vi "Save Section Datas.vi"(8 "error in (no error)":errorcluster, 11 "Section in":refnum<data-value>) -> (0 "error out":errorcluster, 2 "Data":string, 3 "Section out":refnum<data-value>)   [LabVIEW 2013, in "Hierarchy Framework.lvlib" / "Section.lvclass"]
uses:
  Section.lvclass
  Item/Item.lvclass
  Channel/Channel.lvclass
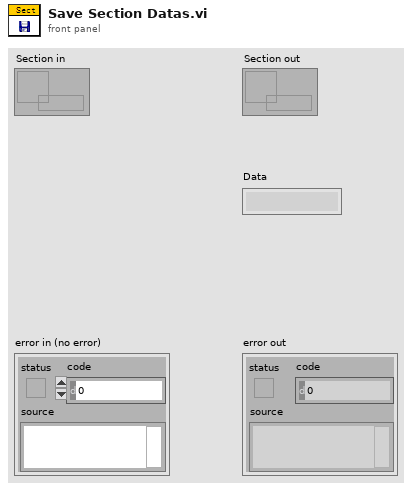
[diagram p1: front panel]
types:
  T1 = typedef "Hierarchy Framework.lvlib/Channel.lvclass/Dimensions.ctl" = cluster{"Row":i32, "Column":i32}
  T2 = typedef "Hierarchy Framework.lvlib/Channel.lvclass/IOType.ctl" = enum16{"Input", "Output"}
  T3 = typedef "Hierarchy Framework.lvlib/Channel.lvclass/Type.ctl" = enum16{"S_Channel", "S_M_Parameter", "S_M_Signal"}
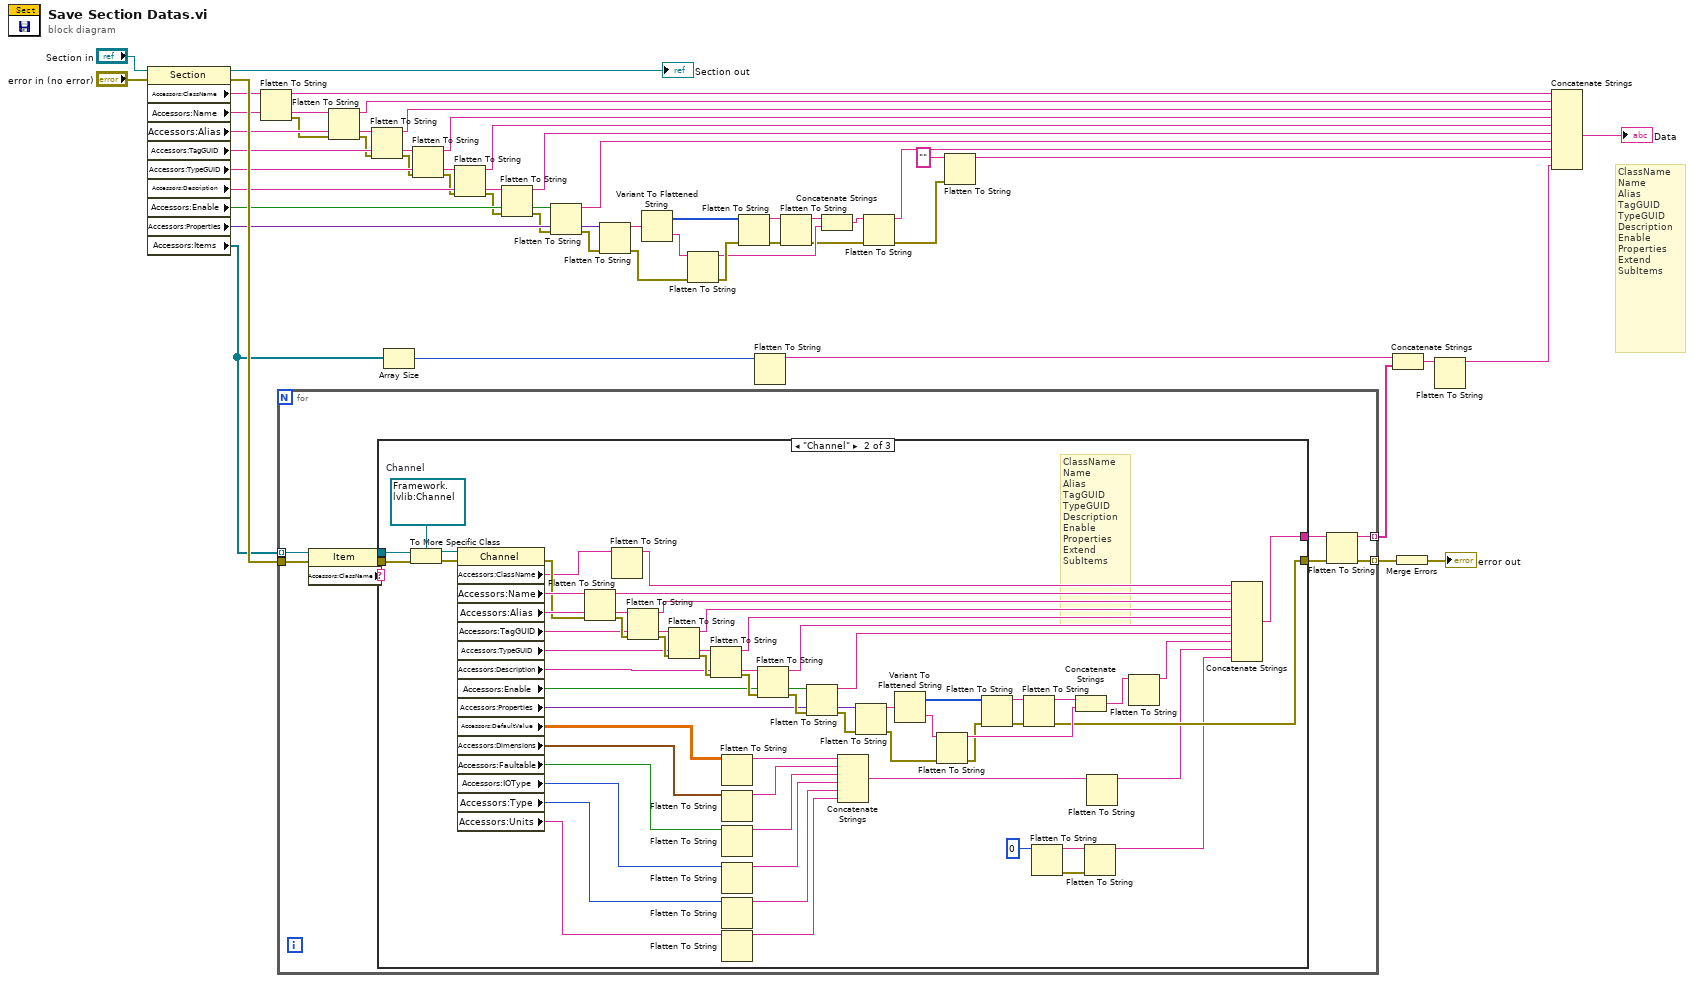
[diagram p0: block diagram]
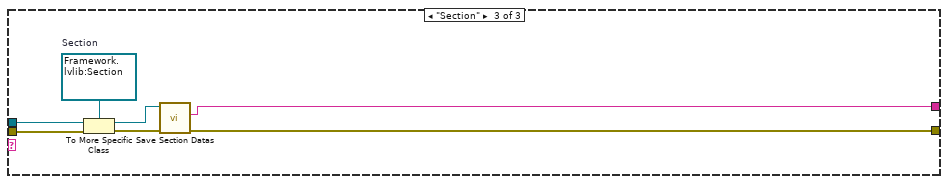
[diagram p3: hidden frame]
diagram:
  # "ClassName\nName\nAlias\nTagGUID\nTypeGUID\nDescription\nEnable\nProperties\nExtend\nSubItems"
  n1 = property class="Section"(reference="Section in", error in="error in (no error)") -> (reference out=→"Section out":refnum<data-value>, error out=w45:errorcluster, "Accessors:ClassName"=w11:string, "Accessors:Name"=w44:string, "Accessors:Alias"=w43:string, "Accessors:TagGUID"=w42:string, "Accessors:TypeGUID"=w41:string, "Accessors:Description"=w40:string, "Accessors:Enable"=w34:bool, "Accessors:Properties"=w30:variant, "Accessors:Items"=w16:refnum<data-value>[])
  n2 = Flatten To String(anything=w11) -> (data string=w9:string, error out=w10:errorcluster)  [unwired: 3 in, 1 out]
  n3 = for {
    tunnel: w16 -> [w59] mode=indexing
    tunnel: [w51] -> w49 mode=indexing
    tunnel: w45 -> [w56]
    tunnel: [w54] -> w12 mode=indexing
    n4 = property class="Item"(reference=w59, error in=w56) -> (reference out=w58:refnum<data-value>, error out=w57:errorcluster, "Accessors:ClassName"=w55:string)
    n5 = case shown="\"Channel\"" w55 {
      tunnel: w58 -> [_ w118 w125]
      tunnel: w57 -> [w60 w117 w124]
      tunnel: [_ w72 w120] -> w53
      tunnel: [w60 w71 w119] -> w52
      frame Default {
      }
      frame "Channel" {
        w116 = refnum<data-value> refnum  # Channel
        # "ClassName\nName\nAlias\nTagGUID\nTypeGUID\nDescription\nEnable\nProperties\nExtend\nSubItems"
        n6 = To More Specific Class(target class=w116, reference=w118, error in=w117) -> (specific class reference=w87:refnum<data-value>, error out=w88:errorcluster)
        n7 = property class="Channel"(reference=w87, error in=w88) -> (error out=w83:errorcluster, "Accessors:ClassName"=w62:string, "Accessors:Name"=w89:string, "Accessors:Alias"=w90:string, "Accessors:TagGUID"=w91:string, "Accessors:TypeGUID"=w92:string, "Accessors:Description"=w93:string, "Accessors:Enable"=w98:bool, "Accessors:Properties"=w102:variant, "Accessors:DefaultValue"=w86:dbl[][], "Accessors:Dimensions"=w84:T1, "Accessors:Faultable"=w85:bool, "Accessors:IOType"=w81:T2, "Accessors:Type"=w80:T3, "Accessors:Units"=w82:string)  [unwired: 1 out]
        n8 = Flatten To String(anything=w89, error in (no error)=w83) -> (data string=w79:string, error out=w110:errorcluster)  [unwired: 2 in, 1 out]
        n9 = Flatten To String(anything=w62) -> (data string=w70:string)  [unwired: 3 in, 2 out]
        n10 = Flatten To String(anything=w90, error in (no error)=w110) -> (data string=w94:string, error out=w111:errorcluster)  [unwired: 2 in, 1 out]
        n11 = Flatten To String(anything=w91, error in (no error)=w111) -> (data string=w95:string, error out=w112:errorcluster)  [unwired: 2 in, 1 out]
        n12 = Flatten To String(anything=w92, error in (no error)=w112) -> (data string=w96:string, error out=w113:errorcluster)  [unwired: 2 in, 1 out]
        n13 = Flatten To String(anything=w86) -> (data string=w78:string)  [unwired: 3 in, 2 out]
        n14 = Flatten To String(anything=w84) -> (data string=w77:string)  [unwired: 3 in, 2 out]
        n15 = Flatten To String(anything=w85) -> (data string=w76:string)  [unwired: 3 in, 2 out]
        n16 = Flatten To String(anything=w81) -> (data string=w75:string)  [unwired: 3 in, 2 out]
        n17 = Flatten To String(anything=w80) -> (data string=w74:string)  [unwired: 3 in, 2 out]
        n18 = Flatten To String(anything=w82) -> (data string=w73:string)  [unwired: 3 in, 2 out]
        n19 = Flatten To String(anything=w93, error in (no error)=w113) -> (data string=w97:string, error out=w114:errorcluster)  [unwired: 2 in, 1 out]
        n20 = Flatten To String(anything=w98, error in (no error)=w114) -> (data string=w99:string, error out=w115:errorcluster)  [unwired: 2 in, 1 out]
        n21 = Concatenate Strings(w78, w77, w76, w75, w74, w73) -> (w69:string)
        n22 = Flatten To String(anything=w102, error in (no error)=w115) -> (data string=w101:string, error out=w106:errorcluster)  [unwired: 2 in, 1 out]
        n23 = Variant To Flattened String(Variant=w101) -> (data string=w103:string, 1:w100:i16[])
        n24 = Flatten To String(anything=w103, error in (no error)=w106) -> (data string=w109:string, error out=w107:errorcluster)  [unwired: 2 in, 1 out]
        n25 = Flatten To String(anything=w100, error in (no error)=w107) -> (data string=w105:string, error out=w104:errorcluster)  [unwired: 2 in, 1 out]
        n26 = Flatten To String(anything=w105, error in (no error)=w104) -> (data string=w108:string, error out=w71:errorcluster)  [unwired: 2 in, 1 out]
        n27 = Flatten To String(anything=0 ("大小")) -> (data string=w66:string, error out=w61:errorcluster)  [unwired: 3 in, 1 out]
        n28 = Concatenate Strings(w108, w109) -> (w64:string)
        n29 = Flatten To String(anything=w66, error in (no error)=w61) -> (data string=w65:string)  [unwired: 2 in, 2 out]
        n30 = Flatten To String(anything=w69) -> (data string=w68:string)  [unwired: 3 in, 2 out]
        n31 = Flatten To String(anything=w64) -> (data string=w63:string)  [unwired: 3 in, 2 out]
        n32 = Concatenate Strings(w70, w79, w94, w95, w96, w97, w99, w63, w68, w65) -> (w72:string)
      }
      frame "Section" {
        w123 = refnum<data-value> refnum  # Section
        n33 = To More Specific Class(target class=w123, reference=w125, error in=w124) -> (specific class reference=w122:refnum<data-value>, error out=w121:errorcluster)
        n34 = call "Save Section Datas.vi"("error in (no error)"=w121, "Section in"=w122) -> ("error out"=w119:errorcluster, "Data"=w120:string)  [unwired: 7 in, 1 out]
      }
    }
    n35 = Flatten To String(anything=w53, error in (no error)=w52) -> (data string=w54:string, error out=w51:errorcluster)  [unwired: 2 in, 1 out]
  }
  n36 = Flatten To String(anything=w44, error in (no error)=w10) -> (data string=w39:string, error out=w22:errorcluster)  [unwired: 2 in, 1 out]
  n37 = Flatten To String(anything=w43, error in (no error)=w22) -> (data string=w38:string, error out=w21:errorcluster)  [unwired: 2 in, 1 out]
  n38 = Array Size(array=w16) -> (size(s)=w15:i32)
  n39 = Flatten To String(anything=w42, error in (no error)=w21) -> (data string=w37:string, error out=w20:errorcluster)  [unwired: 2 in, 1 out]
  n40 = Flatten To String(anything=w41, error in (no error)=w20) -> (data string=w36:string, error out=w19:errorcluster)  [unwired: 2 in, 1 out]
  n41 = Flatten To String(anything=w40, error in (no error)=w19) -> (data string=w35:string, error out=w18:errorcluster)  [unwired: 2 in, 1 out]
  n42 = Flatten To String(anything=w34, error in (no error)=w18) -> (data string=w33:string, error out=w17:errorcluster)  [unwired: 2 in, 1 out]
  n43 = Flatten To String(anything=w30, error in (no error)=w17) -> (data string=w31:string, error out=w26:errorcluster)  [unwired: 2 in, 1 out]
  n44 = Variant To Flattened String(Variant=w31) -> (data string=w29:string, 1:w32:i16[])
  n45 = Flatten To String(anything=w29, error in (no error)=w26) -> (data string=w23:string, error out=w25:errorcluster)  [unwired: 2 in, 1 out]
  n46 = Flatten To String(anything=w32, error in (no error)=w25) -> (data string=w27:string, error out=w28:errorcluster)  [unwired: 2 in, 1 out]
  n47 = Flatten To String(anything=w15) -> (data string=w14:string)  [unwired: 3 in, 2 out]
  n48 = Flatten To String(anything=w27, error in (no error)=w28) -> (data string=w24:string, error out=w2:errorcluster)  [unwired: 2 in, 1 out]
  n49 = Concatenate Strings(w24, w23) -> (w4:string)
  n50 = Flatten To String(anything=w4, error in (no error)=w2) -> (data string=w3:string, error out=w1:errorcluster)  [unwired: 2 in, 1 out]
  n51 = Flatten To String(anything="" ("字符串"), error in (no error)=w1) -> (data string=w7:string)  [unwired: 2 in, 2 out]
  n52 = Concatenate Strings(w14, w12) -> (w13:string)
  n53 = Merge Errors(w49) -> (→"error out":errorcluster)
  n54 = Flatten To String(anything=w13) -> (data string=w6:string)  [unwired: 3 in, 2 out]
  n55 = Concatenate Strings(w9, w39, w38, w37, w36, w35, w33, w3, w7, w6) -> (→"Data":string)
